vi "setSerializedData.vi"(0 "reference":refnum<class "InterfaceNode.lvclass">, 1 "parent":refnum<class "AbstractNode.lvclass">, 2 "children":refnum<class "AbstractNode.lvclass">[](array[class]), 3 "xmlOut":string, 5 "error in (no error)":errorcluster) -> (14 "reference out":refnum<class "InterfaceNode.lvclass">, 19 "error out":errorcluster)   [LabVIEW 2014, in "InterfaceNode.lvclass"]
doc: "setSerializedData"
uses:
  <resource>/Framework/Providers/Open_GDS/UML/InterfaceNode_class/InterfaceNode.lvclass
  <resource>/Framework/Providers/Open_GDS/UML/AbstractNode_class/AbstractNode.lvclass
  <resource>/Framework/Providers/Open_GDS/UML/General/Rectangle/Rectangle Rectangle2D.ctl
  <resource>/Framework/Providers/Open_GDS/UML/MultiLineString_class/MultiLineString.lvclass
  <resource>/Framework/Providers/Open_GDS/UML/RectangularNode_class/RectangularNode.lvclass
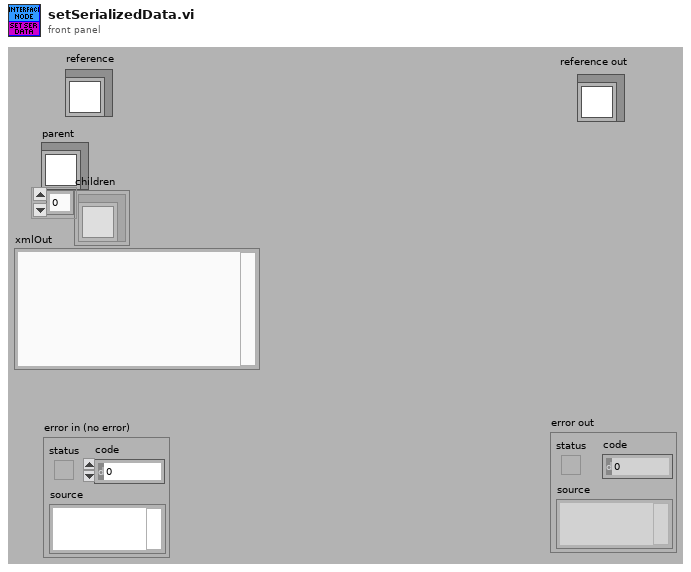
[diagram p1: front panel]
types:
  T1 = typedef "Rectangle Rectangle2D.ctl" = cluster{"x":dbl, "y":dbl, "width":dbl, "height":dbl}
  T2 = cluster{"Base class":cluster{"Base class":cluster{"parent":refnum<k1>, "children":refnum<k1>[], "Hidden":bool}, "bounds":T1}, "midHeight":dbl, "botHeight":dbl, "name":refnum<k1>, "methods":refnum<k1>, "DEFAULT_COMPARTMENT_HEIGHT":i32, "DEFAULT_WIDTH":i32, "DEFAULT_HEIGHT":i32}
  T3 = cluster{"Attributes":cluster{"Base class":cluster{"Base class":cluster{"parent":refnum<k1>, "children":refnum<k1>[], "Hidden":bool}, "bounds":T1}, "midHeight":dbl, "botHeight":dbl, "name":refnum<k1>, "methods":refnum<k1>, "DEFAULT_COMPARTMENT_HEIGHT":i32, "DEFAULT_WIDTH":i32, "DEFAULT_HEIGHT":i32}, string, string}
  T4 = typedef "InterfaceNode.lvclass/ObjectAttributes.ctl" = cluster{"midHeight":dbl, "botHeight":dbl, "name":refnum<class "MultiLineString.lvclass">, "methods":refnum<class "MultiLineString.lvclass">, "DEFAULT_COMPARTMENT_HEIGHT":i32, "DEFAULT_WIDTH":i32, "DEFAULT_HEIGHT":i32}
  T5 = typedef "RectangularNode.lvclass/ObjectAttributes.ctl" = cluster{"bounds":T1}
  T6 = typedef "AbstractNode.lvclass/ObjectAttributes.ctl" = cluster{"parent":refnum<class "AbstractNode.lvclass">, "children":refnum<class "AbstractNode.lvclass">[], "Hidden":bool}
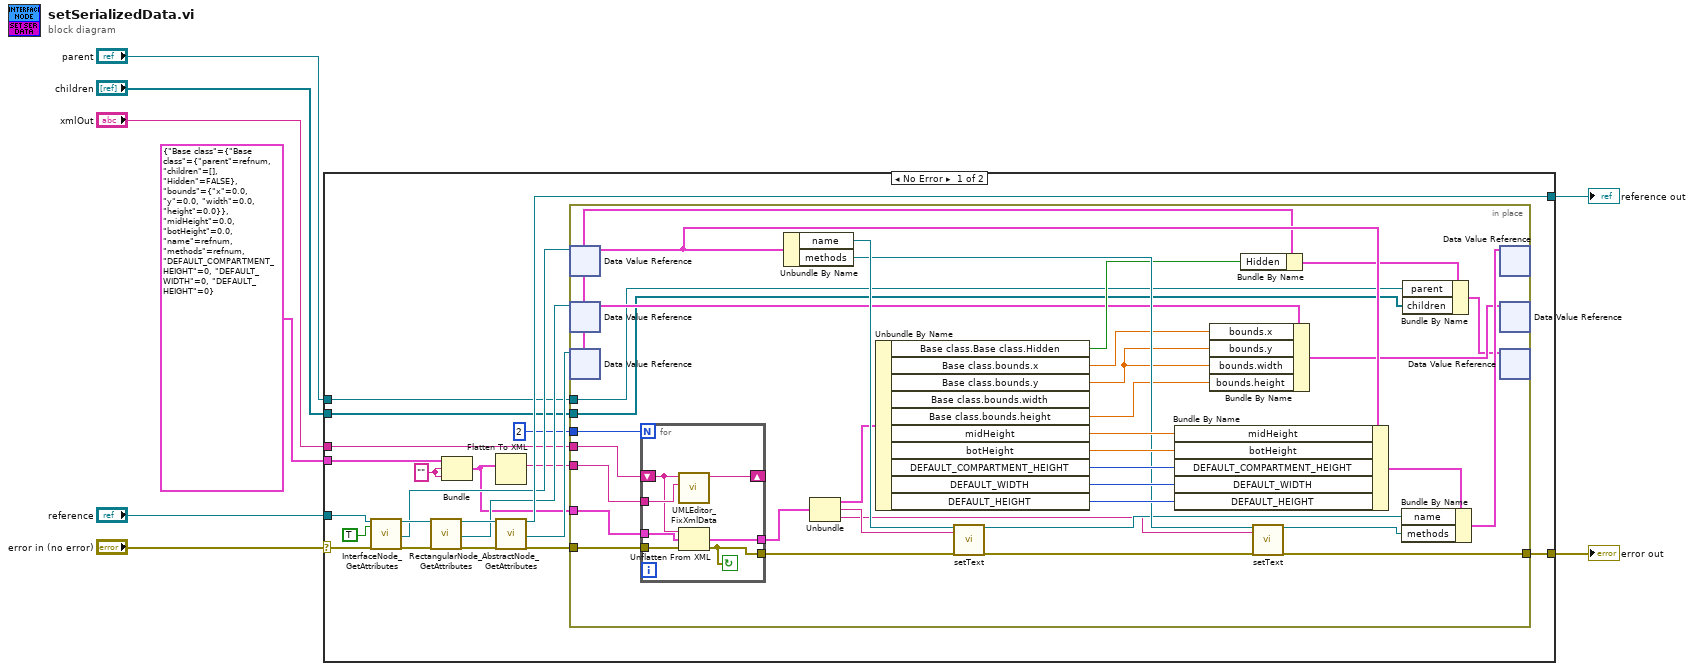
[diagram p0: block diagram]
diagram:
  n1 = case shown="No Error" "error in (no error)" {
    selector: "error in (no error)" -> [w28 w72]
    tunnel: "reference" -> [w29 w73]
    tunnel: [w27 w72] -> w6
    tunnel: [w25 w73] -> w5
    tunnel: "xmlOut" -> [w11 _]
    tunnel: "parent" -> [w10 _]
    tunnel: "children" -> [w9 _]
    tunnel: T2 {"Base class"={"Base class"={"parent"=refnum, "children"=[], "Hidden"=FALSE}, "bounds"={"x"=0.0, "y"=0.0, "width"=0.0, "height"=0.0}}, "midHeight"=0.0, "botHeight"=0.0, "name"=refnum, "methods"=refnum, "DEFAULT_COMPARTMENT_HEIGHT"=0, "DEFAULT_WIDTH"=0, "DEFAULT_HEIGHT"=0} ("Attributes") -> [w24 _]
    frame No Error {
      w26 = ""
      n2 = call <resource>:"InterfaceNode_GetAttributes.vi"("reference in"=w29, "OnlyGetDvrReference(False)"=TRUE, "error in (no error)"=w28) -> ("reference out"=w22:refnum<class "InterfaceNode.lvclass">, "DataRef"=w18:refnum<data-value>, "error out"=w21:errorcluster)  [unwired: 13 in, 1 out]
      n3 = call <resource>:"RectangularNode_GetAttributes.vi"("reference in"=w22, "error in (no error)"=w21) -> ("reference out"=w20:refnum<class "InterfaceNode.lvclass">, "DataRef"=w17:refnum<data-value>, "error out"=w19:errorcluster)  [unwired: 14 in, 1 out]
      n4 = Bundle("Attributes"=w24, w26, w26) -> (w12:T3)  [unwired: 1 out]
      n5 = Flatten To XML(anything=w12) -> (xml string=w13:string)
      n6 = call <resource>:"AbstractNode_GetAttributes.vi"("reference in"=w20, "error in (no error)"=w19) -> ("reference out"=w25:refnum<class "InterfaceNode.lvclass">, "DataRef"=w16:refnum<data-value>, "error out"=w14:errorcluster)  [unwired: 14 in, 1 out]
      n7 = in-place {
        in-place-border: [w43] -> w27
        in-place-border: 2 -> [w38]
        in-place-border: w14 -> [w37]
        in-place-border: w13 -> [w36]
        in-place-border: w12 -> [w35]
        in-place-border: w11 -> [w34]
        in-place-border: w10 -> [w33]
        in-place-border: w9 -> [w32]
        n8 = in-place-dvr #1(w18) -> (w64:T4)  [unwired: 1 out]
        n9 = in-place-dvr #2(w17) -> (w39:T5)  [unwired: 1 out]
        n10 = in-place-dvr #3(w16) -> (w41:T6)  [unwired: 1 out]
        n11 = for {
          N: w38 -> [_]
          tunnel: w37 -> [w71]
          tunnel: [w67] -> w46
          tunnel: [w70] -> w42
          tunnel: w36 -> [w69]
          tunnel: w35 -> [w68]
          shift-right: [w66] -> _
          shift-left: w34 -> [w65]
          stop <- w67 continue-if-true
          n12 = call <resource>:"UMLEditor_FixXmlData.vi"("XmlTemplateIn"=w69, "xmlIn"=w65) -> ("XML OUt"=w66:string)  [unwired: 9 in]
          n13 = Unflatten From XML(xml string=w65, type=w68, error in (no error)=w71) -> (value=w70:T3, error out=w67:errorcluster)
        }
        n14 = Unbundle By Name(w64) -> ("name"=w57:refnum<class "MultiLineString.lvclass">, "methods"=w56:refnum<class "MultiLineString.lvclass">)
        n15 = Unbundle(w42) -> ("Attributes"=w52:T2, w47:string, w44:string)
        n16 = Unbundle By Name(w52) -> ("Base class.Base class.Hidden"=w51:bool, "Base class.bounds.x"=w50:dbl, "Base class.bounds.y"=w49:dbl, "Base class.bounds.height"=w48:dbl, "midHeight"=w63:dbl, "botHeight"=w62:dbl, "DEFAULT_COMPARTMENT_HEIGHT"=w61:i32, "DEFAULT_WIDTH"=w60:i32, "DEFAULT_HEIGHT"=w59:i32)  [unwired: 1 out]
        n17 = call-dynamic "setText.vi"("reference"=w57, "text"=w47, "error in (no error)"=w46) -> ("reference out"=w55:refnum<class "MultiLineString.lvclass">, "error out"=w45:errorcluster)  [unwired: 15 out]
        n18 = Bundle By Name(cluster=w64, "midHeight"=w63, "botHeight"=w62, "DEFAULT_COMPARTMENT_HEIGHT"=w61, "DEFAULT_WIDTH"=w60, "DEFAULT_HEIGHT"=w59) -> (w58:T4)
        n19 = Bundle By Name(cluster=w39, "bounds.x"=w50, "bounds.y"=w49, "bounds.width"=w49, "bounds.height"=w48) -> (w31:T5)
        n20 = Bundle By Name(cluster=w41, "Hidden"=w51) -> (w40:T6)
        n21 = call-dynamic "setText.vi"("reference"=w56, "text"=w44, "error in (no error)"=w45) -> ("reference out"=w54:refnum<class "MultiLineString.lvclass">, "error out"=w43:errorcluster)  [unwired: 15 out]
        n22 = Bundle By Name(cluster=w58, "name"=w55, "methods"=w54) -> (w53:T4)
        n23 = Bundle By Name(cluster=w40, "parent"=w33, "children"=w32) -> (w30:T6)
        n24 = in-place-dvr #1(w53) -> ()  [unwired: 2 out]
        n25 = in-place-dvr #2(w31) -> ()  [unwired: 2 out]
        n26 = in-place-dvr #3(w30) -> ()  [unwired: 2 out]
      }
    }
    frame Error {
    }
  }
  "reference out" <- w5
  "error out" <- w6
